vi "Destroy Writer Endpoint.vi"(8 "error in (no error)":errorcluster, 11 "Stream in":refnum<class "Stream.lvclass">) -> (0 "error out":errorcluster, 3 "Stream out":refnum<class "Stream.lvclass">)   [LabVIEW 2018, in "Stream.lvclass"]
doc: "Destroy writer endpoint"
uses:
  Stream.lvclass
  Stream.lvclass/Stream.ctl
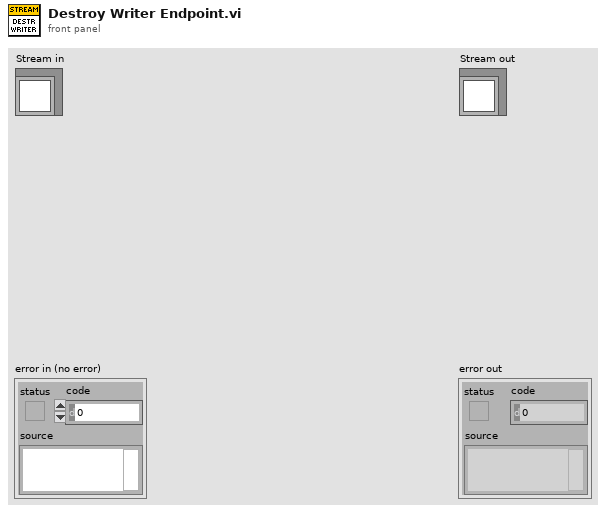
[diagram p1: front panel]
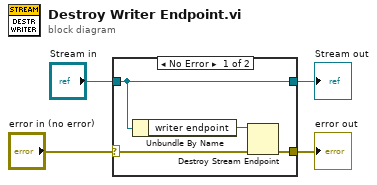
[diagram p0: block diagram]
diagram:
  n1 = case shown="No Error" "error in (no error)" {
    selector: "error in (no error)" -> [w7 w10]
    tunnel: [w8 w10] -> w3
    tunnel: [w6 w9] -> w1
    tunnel: "Stream in" -> [w6 w9]
    frame No Error {
      n2 = Unbundle By Name(w6) -> ("writer endpoint"=w5:refnum<k21>)
      n3 = Destroy Stream Endpoint(8:w7, 11:w5) -> (0:w8:errorcluster)
    }
    frame Error {
    }
  }
  "error out" <- w3
  "Stream out" <- w1
